vi "_JSON.Test2.vi"() -> ()   [LabVIEW 2018]
uses:
  <vilib>/KATE/Time/Time Utils.lvlib
panel:
  out "Duration(s)":dbl
  out "SN":i32
  in  "Path":path
  out "error out":errorcluster
  out "baseCalibration":dbl[](array[numeric])
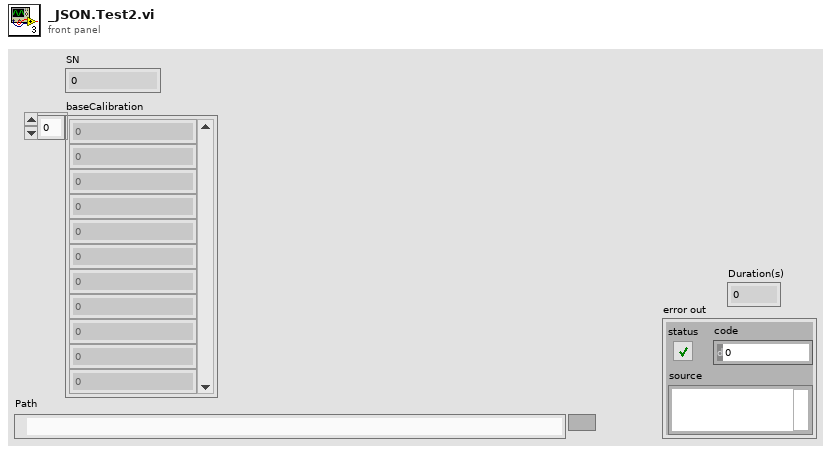
[diagram p1: front panel]
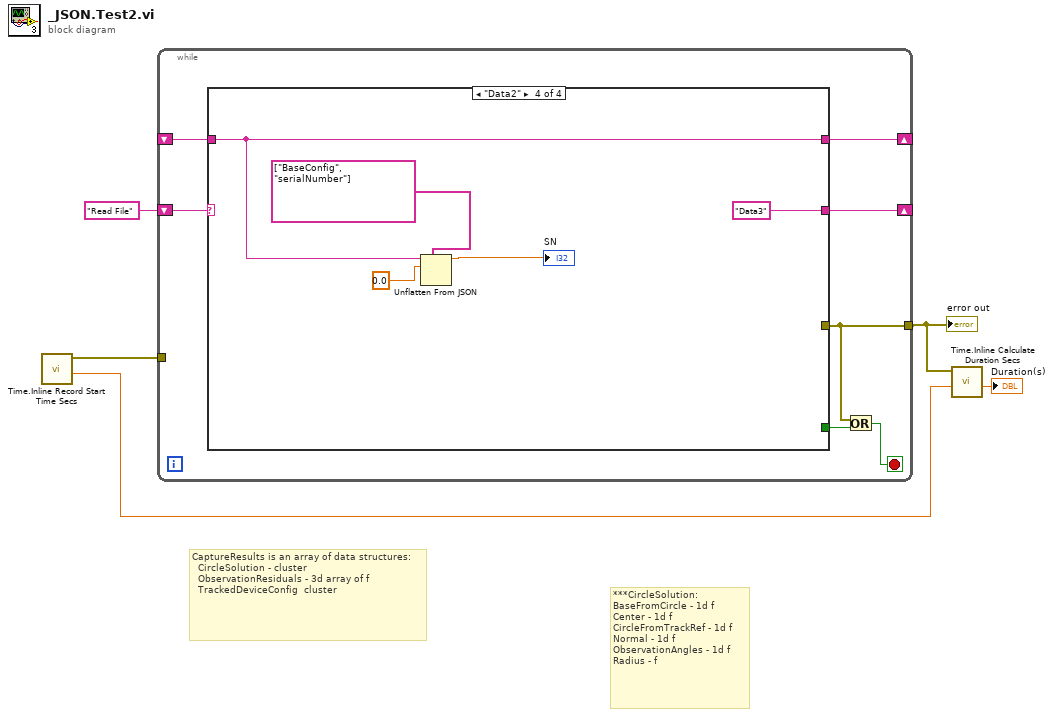
[diagram p0: block diagram]
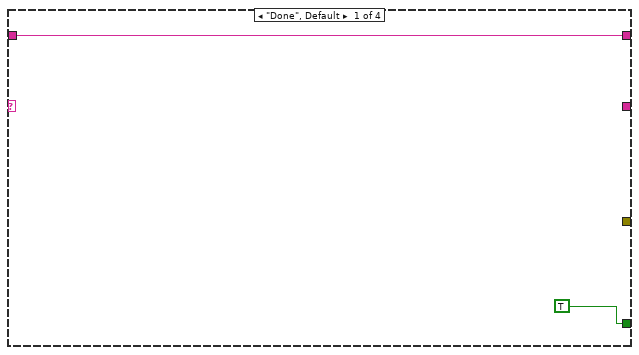
[diagram p2: hidden frame]
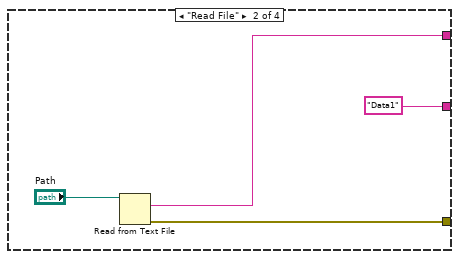
[diagram p3: hidden frame]
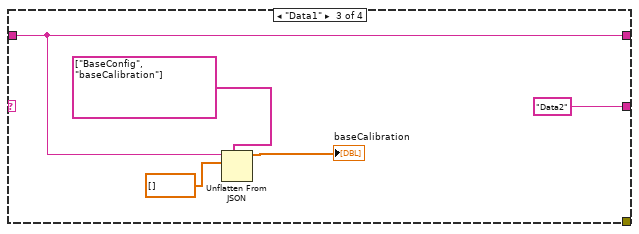
[diagram p4: hidden frame]
diagram:
  # "***CircleSolution:\nBaseFromCircle - 1d f\nCenter - 1d f\nCircleFromTrackRef - 1d f\nNormal - 1d f\nObservationAngles - 1d f\nRadius - f"
  # "CaptureResults is an array of data structures:\n  CircleSolution - cluster\n  ObservationResiduals - 3d array of f\n  TrackedDeviceConfig  cluster"
  n1 = call <vilib>:"Time.Inline Record Start Time Secs.vi"() -> ("Start(s)"=w2:dbl, "Error Out Upper"=w4:errorcluster)  [unwired: 9 in, 1 out]
  n2 = while {
    shift-right: [w7] -> _
    shift-left: _ -> [w11]
    shift-right: [w8] -> _
    shift-left: "Read File" -> [w12]
    tunnel: [w6] -> w3
    tunnel: w4 -> [_]
    stop <- w10 stop-if-true
    n3 = case shown="\"Data2\"" w12 {
      tunnel: w11 -> [w13 _ w19 w26]
      tunnel: [TRUE _ _ _] -> w9
      tunnel: [_ w17 _ _] -> w6
      tunnel: [_ "Data1" "Data2" "Data3"] -> w8
      tunnel: [w13 w15 w19 w26] -> w7
      frame "Done", Default {
      }
      frame "Read File" {
        n4 = Read from Text File(file (use dialog)="Path") -> (text=w15:string, error out=w17:errorcluster)  [unwired: 3 in, 2 out]
      }
      frame "Data1" {
        n5 = Unflatten From JSON(path=string[] ["BaseConfig", "baseCalibration"], JSON string=w19, type and defaults=dbl[] [] ("Data")) -> (value=→"baseCalibration":dbl[])  [unwired: 4 in, 1 out]
      }
      frame "Data2" {
        n6 = Unflatten From JSON(path=string[] ["BaseConfig", "serialNumber"], JSON string=w26, type and defaults=0.0) -> (value=→"SN":dbl)  [unwired: 4 in, 1 out]
      }
    }
    n7 = Or(x=w6, y=w9) -> (x .or. y?=w10:bool)
  }
  "error out" <- w3
  n8 = call <vilib>:"Time.Inline Calculate Duration Secs.vi"("Start(Sec)"=w2, "Error In Top"=w3) -> ("Duration(s)"=→"Duration(s)":dbl)  [unwired: 7 in, 2 out]
